vi "Load File.vi"(5 "...to scan":i32, 6 "Channels":string[](array[string]), 7 "from scan...":i32, 8 "error in (no error)":errorcluster, 9 "Other channels":string[](array[string]), 10 "File Path":path, 11 "dIdV State in":refnum<class "Point Contact Model.lvclass">) -> (0 "error out":errorcluster, 1 "Other values":string[](array[string]), 2 "Number of scans":i32, 3 "dIdV State out":refnum<class "Point Contact Model.lvclass">)   [LabVIEW 2021, in "Point Contact Model.lvclass"]
uses:
  Point Contact Model.lvclass
  Point Contact Model.lvclass/Point Contact Model.ctl
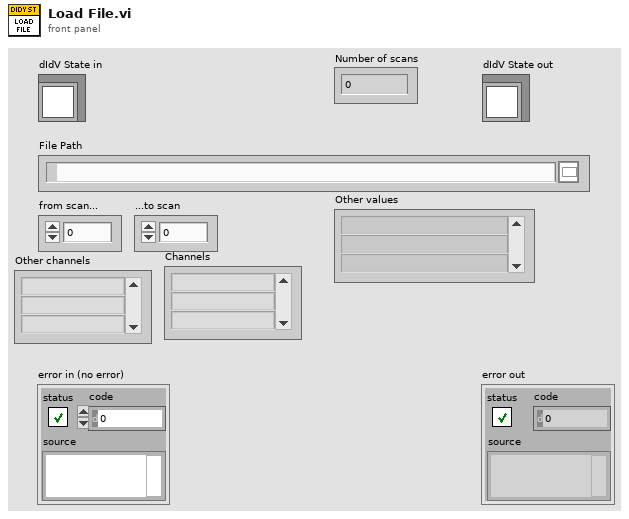
[diagram p1: front panel]
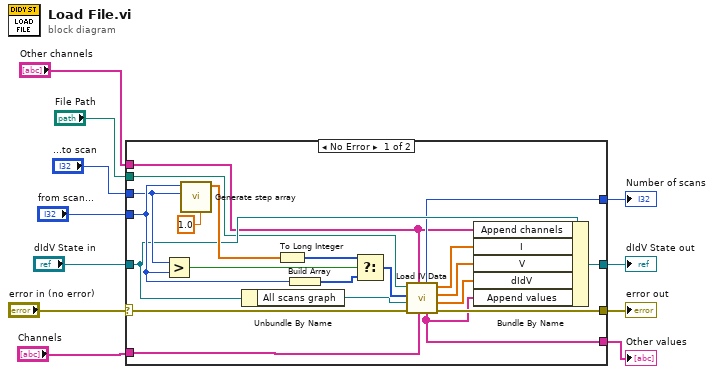
[diagram p0: block diagram]
diagram:
  n1 = case shown="No Error" "error in (no error)" {
    selector: "error in (no error)" -> [w22 w34]
    tunnel: [w21 w34] -> w10
    tunnel: [w20 w33] -> w8
    tunnel: "dIdV State in" -> [w24 w33]
    tunnel: "from scan..." -> [w26 _]
    tunnel: "...to scan" -> [w25 _]
    tunnel: "File Path" -> [w16 _]
    tunnel: [w15 _] -> w4
    tunnel: [w13 _] -> w3
    tunnel: "Other channels" -> [w14 _]
    tunnel: "Channels" -> [w12 _]
    frame No Error {
      n2 = Greater?(x=w25, y=w26) -> (0:w29:bool)
      n3 = call "Generate step array.vi"("Step"=1.0, "End"=w25, "Start"=w26) -> ("Steps"=w30:dbl[])  [unwired: 8 in]
      n4 = Unbundle By Name(w24) -> ("All scans graph"=w23:refnum<vi>)
      n5 = To Long Integer(number=w30) -> (32bit integer=w27:i32[])
      n6 = Build Array(w26) -> (w28:i32[])
      n7 = Select(t=w27, s=w29, f=w28) -> (s? t:f=w32:i32[])
      n8 = call "Load IV Data.vi"("Channels"=w12, "Other channels"=w14, "error in"=w22, "All scans"=w23, "Scan numbers"=w32, "File Path"=w16) -> ("error out"=w21:errorcluster, "dIdV"=w17:dbl[], "V"=w18:dbl[], "I"=w19:dbl[], "Other values"=w13:string[], "Number of scans"=w15:i32)
      n9 = Bundle By Name(cluster=w24, "Append channels"=w14, "I"=w19, "V"=w18, "dIdV"=w17, "Append values"=w13) -> (w20:refnum<class "Point Contact Model.lvclass">)
    }
    frame Error {
    }
  }
  "error out" <- w10
  "dIdV State out" <- w8
  "Number of scans" <- w4
  "Other values" <- w3
